vi "Reserve I2C.vi"(7 "I2C Pins":T1={"SDA GPIO"=-1, "SCL GPIO"=-1}, 8 "error in (no error)":errorcluster, 9 "Purpose":string, 10 "I2C #":T3=-1, 11 "Session in":refnum<class "Session.lvclass">) -> (0 "error out":errorcluster, 3 "Session out":refnum<class "Session.lvclass">)   [LabVIEW 2024, in "CTI.lvlib" / "Session.lvclass"]
uses:
  Session.lvclass
  I2C Number.ctl
  I2C Pins.ctl
  GPIO Number.ctl
  Resource/Resource.lvclass/Resource.ctl
  Session.lvclass/Session.ctl
  dcef0d26-6755-4235-b060-6b0e00c3d74f.vi
  dcef0d26-6755-4235-b060-6b0e00c3d74f.vi/685f7f19-b444-4620-8f66-e6e2ddd64bb8.vi
  I2C/I2C.lvclass
  C:/Users/nkirchne/Documents/~SANDBOX/Electronics Workflow/build/ForPort/CTI/Resource/Resource.lvclass
  Generate Error.vi
  Resource/Resource.lvclass
  CTI.lvlib
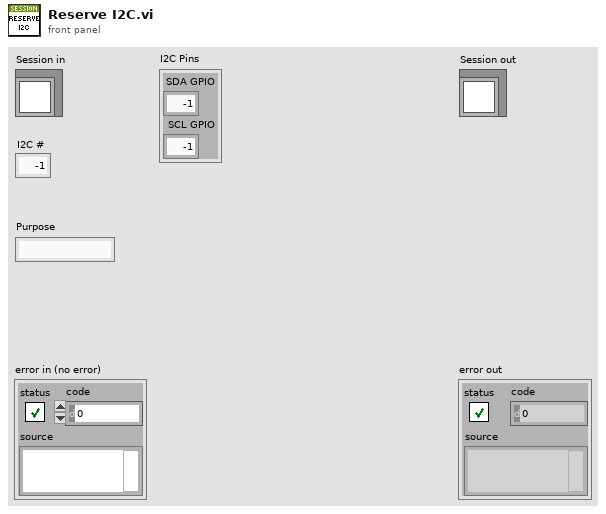
[diagram p1: front panel]
types:
  T1 = typedef "CTI.lvlib/I2C Pins.ctl" = cluster{"SDA GPIO":T2, "SCL GPIO":T2}
  T2 = typedef "CTI.lvlib/GPIO Number.ctl" = i8
  T3 = typedef "CTI.lvlib/I2C Number.ctl" = i8
  T4 = typedef "CTI.lvlib/Session.lvclass/Resources.ctl" = cluster{"GPIO":map{T2, refnum<class "GPIO.lvclass">}, "AI":map{T5, refnum<class "AI.lvclass">}, "PWM":map{T2, refnum<class "PWM.lvclass">}, "UART":map{T6, refnum<class "UART.lvclass">}, "I2C":map{T3, refnum<class "I2C.lvclass">}, "SPI":map{T7, refnum<class "SPI.lvclass">}, "SPI CS":map{T2, refnum<class "SPI CS.lvclass">}}
  T5 = typedef "CTI.lvlib/ADC Number.ctl" = i8
  T6 = typedef "CTI.lvlib/UART Number.ctl" = i8
  T7 = typedef "CTI.lvlib/SPI Number.ctl" = i8
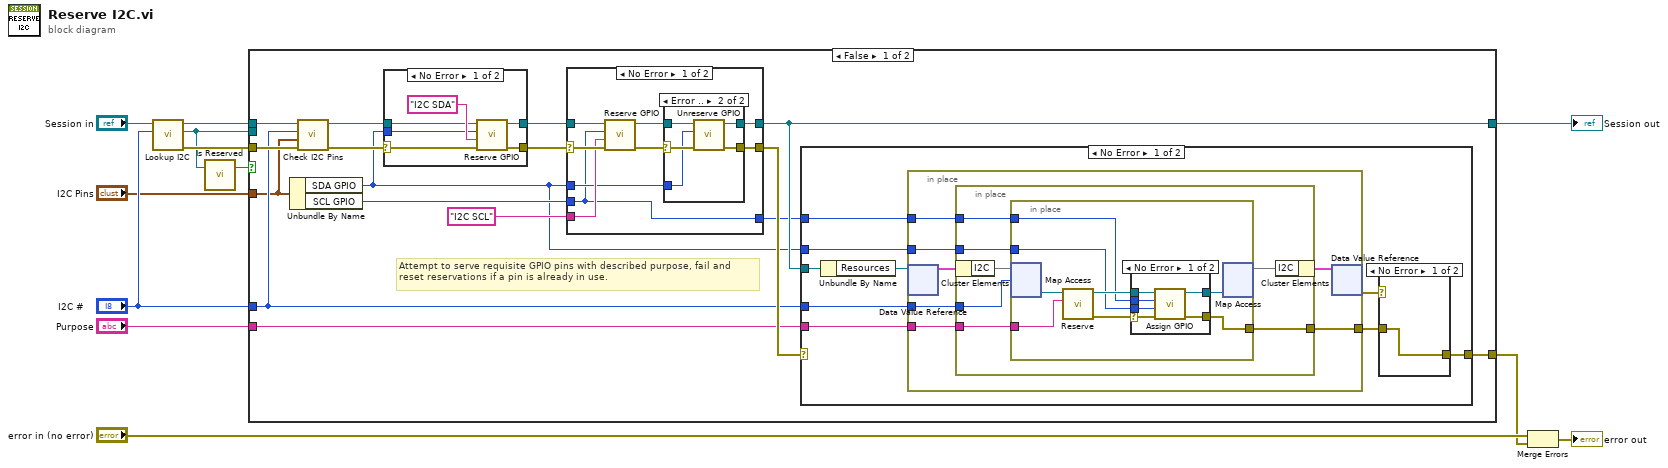
[diagram p0: block diagram]
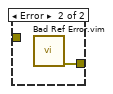
[diagram p6: hidden frame]
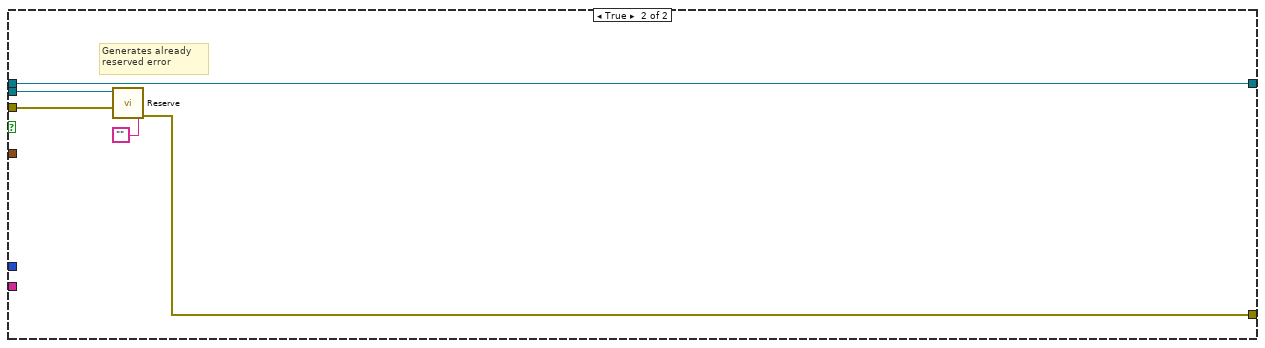
[diagram p8: hidden frame]
diagram:
  n1 = call "Lookup I2C.vi"("I2C #"="I2C #", "Session in"="Session in") -> ("error out"=w12:errorcluster, "I2C"=w1:refnum<class "I2C.lvclass">, "Session out"=w6:refnum<class "Session.lvclass">)  [unwired: 7 in]
  n2 = call "Is Reserved.vi"("Resource in"=w1) -> ("Reserved"=w2:bool)  [unwired: 6 in]
  n3 = case shown="False" w2 {
    tunnel: w12 -> [w25 w100]
    tunnel: "Purpose" -> [w24 _]
    tunnel: [w23 w98] -> w7
    tunnel: w6 -> [w17 w99]
    tunnel: "I2C #" -> [w15 _]
    tunnel: "I2C Pins" -> [w14 _]
    tunnel: [w21 w99] -> w3
    tunnel: w1 -> [_ w101]
    frame False {
      # "Attempt to serve requisite GPIO pins with described purpose, fail and reset reservations if a pin is already in use."
      n4 = Unbundle By Name(w14) -> ("SDA GPIO"=w13:T2, "SCL GPIO"=w20:T2)
      n5 = call "Check I2C Pins.vi"("error in (no error)"=w25, "I2C Pins"=w14, "I2C #"=w15, "Session in"=w17) -> ("error out"=w28:errorcluster, "Session out"=w16:refnum<class "Session.lvclass">)  [unwired: 6 in]
      n6 = case shown="No Error" w28 {
        selector: w28 -> [w30 w35]
        tunnel: [w34 w35] -> w26
        tunnel: [w32 w36] -> w22
        tunnel: w13 -> [w31 _]
        tunnel: w16 -> [w29 w36]
        frame No Error {
          n7 = call "Reserve GPIO.vi"("error in (no error)"=w30, "Purpose"="I2C SDA", "GPIO #"=w31, "Session in"=w29) -> ("error out"=w34:errorcluster, "Session out"=w32:refnum<class "Session.lvclass">)  [unwired: 6 in]
        }
        frame Error {
        }
      }
      n8 = case shown="No Error" w26 {
        selector: w26 -> [w45 w53]
        tunnel: [w39 w53] -> w27
        tunnel: w22 -> [w44 w54]
        tunnel: [w40 w54] -> w21
        tunnel: w20 -> [w37 _]
        tunnel: "I2C SCL" ("Purpose") -> [w43 _]
        tunnel: w13 -> [w38 _]
        tunnel: [w37 _] -> w18
        frame No Error {
          n9 = call "Reserve GPIO.vi"("error in (no error)"=w45, "Purpose"=w43, "GPIO #"=w37, "Session in"=w44) -> ("error out"=w42:errorcluster, "Session out"=w41:refnum<class "Session.lvclass">)  [unwired: 6 in]
          n10 = case shown="Error .." w42 {
            selector: w42 -> [w46 w51]
            tunnel: w41 -> [w47 w52]
            tunnel: [w47 w48] -> w40
            tunnel: [w46 w49] -> w39
            tunnel: w38 -> [_ w50]
            frame No Error {
            }
            frame Error {
              n11 = call "Unreserve GPIO.vi"("error in (no error)"=w51, "GPIO #"=w50, "Session in"=w52) -> ("error out"=w49:errorcluster, "Session out"=w48:refnum<class "Session.lvclass">)  [unwired: 7 in]
            }
          }
        }
        frame Error {
        }
      }
      n12 = case shown="No Error" w27 {
        selector: w27 -> [_ w96]
        tunnel: w24 -> [w62 _]
        tunnel: [w59 w96] -> w23
        tunnel: w15 -> [w58 _]
        tunnel: w21 -> [w57 _]
        tunnel: w18 -> [w56 _]
        tunnel: w13 -> [w55 _]
        frame No Error {
          n13 = Unbundle By Name(w57) -> ("Resources"=w63:refnum<data-value>)
          n14 = in-place {
            in-place-border: w58 -> [w70]
            in-place-border: w62 -> [w69]
            in-place-border: [w68] -> w61
            in-place-border: w56 -> [w65]
            in-place-border: w55 -> [w64]
            n15 = in-place-dvr #1(w63) -> (w66:T4)  [unwired: 1 out]
            n16 = in-place {
              in-place-border: w70 -> [w76]
              in-place-border: w69 -> [w75]
              in-place-border: [w74] -> w68
              in-place-border: w65 -> [w72]
              in-place-border: w64 -> [w71]
              n17 = in-place-cluster #2(w66) -> ("I2C"=w77:map{T3, refnum<class "I2C.lvclass">})
              n18 = in-place {
                in-place-border: w75 -> [w84]
                in-place-border: [w78] -> w74
                in-place-border: w72 -> [w81]
                in-place-border: w71 -> [w80]
                n19 = in-place-map #3(w77, w76) -> (w85:refnum<class "I2C.lvclass">)  [unwired: 1 in, 1 out]
                n20 = call "Reserve.vi"("Purpose"=w84, "Resource in"=w85) -> ("error out"=w79:errorcluster, "Resource out"=w83:refnum<class "I2C.lvclass">)  [unwired: 8 in]
                n21 = case shown="No Error" w79 {
                  selector: w79 -> [w87 w93]
                  tunnel: w83 -> [w91 w92]
                  tunnel: [w90 w92] -> w82
                  tunnel: w81 -> [w89 _]
                  tunnel: w80 -> [w88 _]
                  tunnel: [w86 w93] -> w78
                  frame No Error {
                    n22 = call "Assign GPIO.vi"("error in (no error)"=w87, "SDA"=w88, "SCL"=w89, "I2C in"=w91) -> ("error out"=w86:errorcluster, "I2C out"=w90:refnum<class "I2C.lvclass">)  [unwired: 6 in]
                  }
                  frame Error {
                  }
                }
                n23 = in-place-map #3(w82) -> (w73:map{T3, refnum<class "I2C.lvclass">})  [unwired: 1 in, 2 out]
              }
              n24 = in-place-cluster #2("I2C"=w73) -> (w67:T4)
            }
            n25 = in-place-dvr #1(w67) -> (w60:errorcluster)  [unwired: 1 out]
          }
          n26 = case shown="No Error" w60 {
            tunnel: w61 -> [w94 _]
            tunnel: [w94 w95] -> w59
            frame No Error {
            }
            frame Error {
              n27 = call "Bad Ref Error.vim"() -> ("error out"=w95:errorcluster)  [unwired: 10 in, 1 out]
            }
          }
        }
        frame Error {
          # "Error generated reserving GPIO Pin(s) or looking up I2C #"
        }
      }
    }
    frame True {
      # "Generates already reserved error"
      n28 = call "Reserve.vi"("error in (no error)"=w100, "Purpose"="", "Resource in"=w101) -> ("error out"=w98:errorcluster)  [unwired: 7 in, 1 out]
    }
  }
  "Session out" <- w3
  n29 = Merge Errors("error in (no error)", w7) -> (→"error out":errorcluster)
